vi "Get Transfer Groups.vi"(11 "Transceiver Thread in":refnum<class "Plugin Thread.lvclass">) -> (2 "Transfer Groups":refnum<class "Transfer Group.lvclass">[](array[class]), 3 "Transceiver Thread out":refnum<class "Plugin Thread.lvclass">)   [LabVIEW 2017, in "DSF Core.lvlib" / "Plugin Thread.lvclass"]
uses:
  Plugin Thread.lvclass
  Transfer Group/Transfer Group.lvclass
  Plugin Thread.lvclass/Plugin Thread.ctl
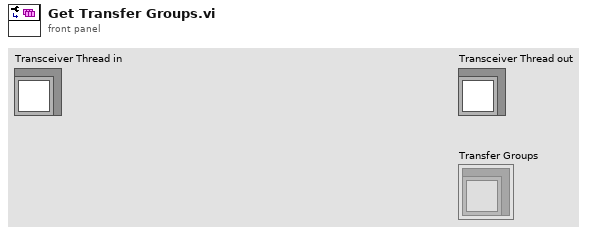
[diagram p1: front panel]
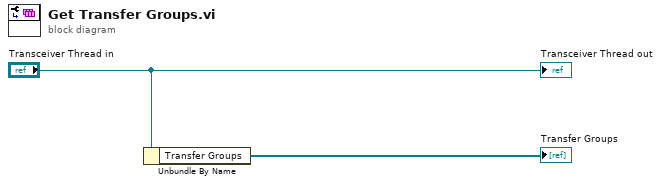
[diagram p0: block diagram]
diagram:
  n1 = Unbundle By Name("Transceiver Thread in") -> ("Transfer Groups"=→"Transfer Groups":refnum<class "Transfer Group.lvclass">[])
  "Transceiver Thread out" <- "Transceiver Thread in"
